vi "Local F310.vi"(8 "error in (no error)":errorcluster, 10 "Deadzone Scale Cluster":cluster{"Scale":dbl, "Deadzone":dbl}, 11 "device ID":refnum<k1>) -> (0 "error out":errorcluster, 1 "Right Stick":cluster{"X":dbl, "Y":dbl}, 2 "Left Stick":cluster{"X":dbl, "Y":dbl}, 3 "device ID":refnum<k1>, 4 "Buttons":T2, 5 "D-Pad":cluster{"X":dbl, "Y":dbl})   [LabVIEW 2013]
uses:
  <vilib>/Utility/inputDevices.llb/joystickAcquire.vi
panel:
  out "D-Pad Buttons":T1
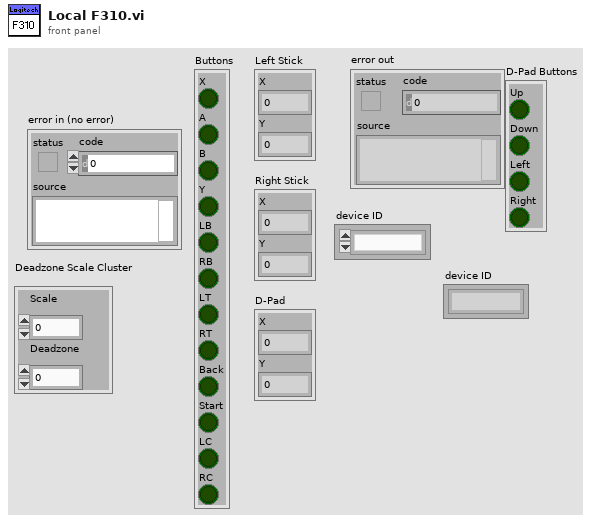
[diagram p1: front panel]
types:
  T1 = cluster{"Up":bool, "Down":bool, "Left":bool, "Right":bool}
  T2 = cluster{"X":bool, "A":bool, "B":bool, "Y":bool, "LB":bool, "RB":bool, "LT":bool, "RT":bool, "Back":bool, "Start":bool, "LC":bool, "RC":bool}
  T3 = cluster{"X axis":i32, "Y axis":i32, "Z axis":i32, "X axis rotation":i32, "Y axis rotation":i32, "Z axis rotation":i32, "U axis":i32, "V axis":i32}
  T4 = cluster{"button 1":bool, "button 2":bool, "button 3":bool, "button 4":bool, "button 5":bool, "button 6":bool, "button 7":bool, "button 8":bool, "button 9":bool, "button 10":bool, "button 11":bool, "button 12":bool, "button 13":bool, "button 14":bool, "button 15":bool, "button 16":bool, "button 17":bool, "button 18":bool, "button 19":bool, "button 20":bool, "button 21":bool, "button 22":bool, "button 23":bool, "button 24":bool, "button 25":bool, "button 26":bool, "button 27":bool, "button 28":bool, "button 29":bool, "button 30":bool, "button 31":bool, "button 32":bool}
  T5 = cluster{"[0]":dbl, "[1]":dbl, "[2]":dbl, "[3]":dbl, "[4]":dbl, "[5]":dbl}
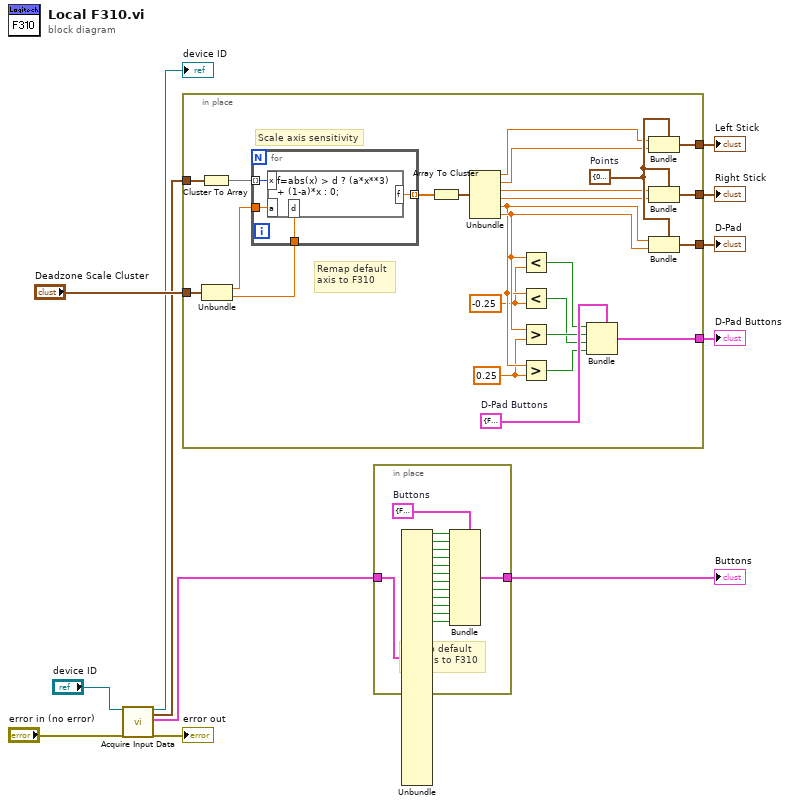
[diagram p0: block diagram]
diagram:
  n1 = call-poly <vilib>:"Acquire Input Data.vi"("device ID"="device ID", "error in (no error)"="error in (no error)") -> ("device ID"=→"device ID":refnum<k1>, "axis info"=w2:T3, "button info"=w1:T4, "error out"=→"error out":errorcluster)  [unwired: 13 in, 1 out]
  n2 = in-place {
    in-place-border: w2 -> [w19]
    in-place-border: [w37] -> w12
    in-place-border: [w36] -> w11
    in-place-border: [w34] -> w10
    in-place-border: [w28] -> w8
    in-place-border: "Deadzone Scale Cluster" -> [w15]
    w29 = -0.25 ("y")
    w30 = 0.25 ("y")
    w33 = T1 {"Up"=FALSE, "Down"=FALSE, "Left"=FALSE, "Right"=FALSE}  # D-Pad Buttons
    w35 = cluster{"X":dbl, "Y":dbl} {"X"=0.0, "Y"=0.0}  # Points
    # "Scale axis sensitivity"
    # "Remap default\naxis to F310"
    n3 = Cluster To Array(cluster=w19) -> (array=w17:i32[])
    n4 = Unbundle(w15) -> ("Scale"=w14:dbl, "Deadzone"=w13:dbl)
    n5 = for {
      tunnel: w17 -> [w41] mode=indexing
      tunnel: [w40] -> w16 mode=indexing
      tunnel: w14 -> [w39]
      tunnel: w13 -> [w38]
      n6 = formula code="f=abs(x) > d ? (a*x**3) + (1-a)*x : 0;"("x"=w41, "a"=w39, "d"=w38) -> ("f"=w40:dbl)
    }
    n7 = Array To Cluster(array=w16) -> (cluster=w18:T5)
    n8 = Unbundle(w18) -> ("[0]"=w23:dbl, "[1]"=w22:dbl, "[2]"=w21:dbl, "[3]"=w20:dbl, "[4]"=w31:dbl, "[5]"=w32:dbl)
    n9 = Less?(x=w32, y=w29) -> (x < y?=w26:bool)
    n10 = Less?(x=w31, y=w29) -> (x < y?=w24:bool)
    n11 = Greater?(x=w32, y=w30) -> (0:w27:bool)
    n12 = Greater?(x=w31, y=w30) -> (0:w25:bool)
    n13 = Bundle(cluster=w33, "Up"=w26, "Down"=w27, "Left"=w24, "Right"=w25) -> (w28:T1)
    n14 = Bundle(cluster=w35, "X"=w23, "Y"=w22) -> (w37:cluster{"X":dbl, "Y":dbl})
    n15 = Bundle(cluster=w35, "X"=w21, "Y"=w20) -> (w36:cluster{"X":dbl, "Y":dbl})
    n16 = Bundle(cluster=w35, "X"=w31, "Y"=w32) -> (w34:cluster{"X":dbl, "Y":dbl})
  }
  "Left Stick" <- w12
  "Right Stick" <- w11
  "D-Pad" <- w10
  "D-Pad Buttons" <- w8
  n17 = in-place {
    in-place-border: w1 -> [w56]
    in-place-border: [w42] -> w9
    w55 = T2 {"X"=FALSE, "A"=FALSE, "B"=FALSE, "Y"=FALSE, "LB"=FALSE, "RB"=FALSE, "LT"=FALSE, "RT"=FALSE, "Back"=FALSE, "Start"=FALSE, "LC"=FALSE, "RC"=FALSE}  # Buttons
    # "Remap default\nbuttons to F310"
    n18 = Unbundle(w56) -> ("button 1"=w54:bool, "button 2"=w53:bool, "button 3"=w52:bool, "button 4"=w51:bool, "button 5"=w50:bool, "button 6"=w49:bool, "button 7"=w48:bool, "button 8"=w47:bool, "button 9"=w46:bool, "button 10"=w45:bool, "button 11"=w44:bool, "button 12"=w43:bool)  [unwired: 20 out]
    n19 = Bundle(cluster=w55, "X"=w54, "A"=w53, "B"=w52, "Y"=w51, "LB"=w50, "RB"=w49, "LT"=w48, "RT"=w47, "Back"=w46, "Start"=w45, "LC"=w44, "RC"=w43) -> (w42:T2)
  }
  "Buttons" <- w9
